vi "Close app.vi"(8 "Error in":errorcluster, 11 "App state":T1) -> (0 "Error out":errorcluster, 1 "Close app?":bool, 3 "App state":T1)   [LabVIEW 2020]
uses:
  Typedefs/State.ctl
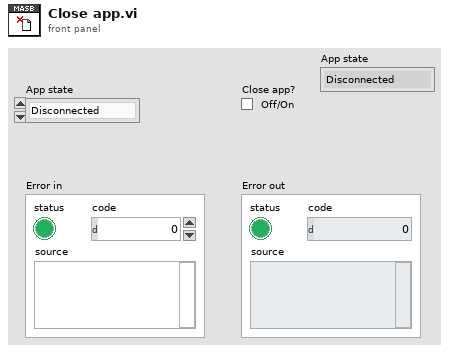
[diagram p1: front panel]
types:
  T1 = typedef "State.ctl" = enum16{"Disconnected", "Connected", "Measuring"}
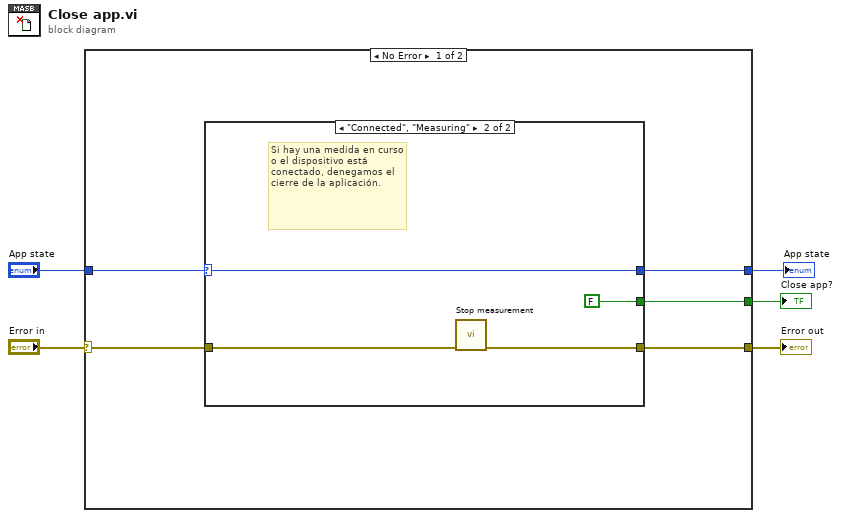
[diagram p0: block diagram]
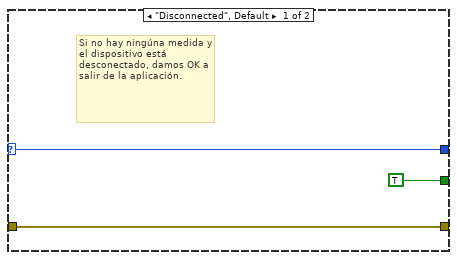
[diagram p2: hidden frame]
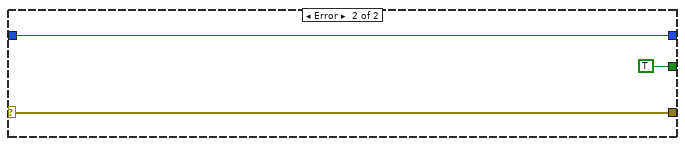
[diagram p3: hidden frame]
diagram:
  n1 = case shown="No Error" "Error in" {
    selector: "Error in" -> [w9 w20]
    tunnel: [w10 TRUE ("Stop")] -> w5
    tunnel: [w8 w20] -> w3
    tunnel: "App state" -> [w7 w18]
    tunnel: [w6 w18] -> w1
    frame No Error {
      n2 = case shown="\"Connected\", \"Measuring\"" w7 {
        selector: w7 -> [w11 w14]
        tunnel: [w13 w17] -> w8
        tunnel: w9 -> [w13 w16]
        tunnel: [TRUE ("Stop") FALSE ("Stop")] -> w10
        tunnel: [w11 w14] -> w6
        frame "Disconnected", Default {
          # "Si no hay ningúna medida y el dispositivo está desconectado, damos OK a salir de la aplicación."
        }
        frame "Connected", "Measuring" {
          # "Si hay una medida en curso o el dispositivo está conectado, denegamos el cierre de la aplicación."
          n3 = call "Stop measurement"("error in (no error)"=w16) -> ("error out"=w17:errorcluster)  [unwired: 9 in, 1 out]
        }
      }
    }
    frame Error {
    }
  }
  "Close app?" <- w5
  "Error out" <- w3
  "App state" <- w1
